vi "resistanceTest.vi"() -> ()   [LabVIEW 2010]
uses:
  <vilib>/DAQmx/read.llb/DAQmx Read (Analog 1D Wfm NChan NSamp).vi
  <vilib>/DAQmx/write.llb/DAQmx Write (Analog DBL 1Chan 1Samp).vi
  <vilib>/daqmx/miscellaneous.llb/DAQmx Fill In Error Info.vi
  <vilib>/ptbypt/NI_PtbyPt.lvlib
panel:
  in  "LowTime":u32
  in  "HighTime":u32
  out "Resistance (MOhm)  2":dbl
  in  "voltage":dbl format="%0.2f"
  out "Test pulse 2":bool
  in  "Test":bool
  out "Numeric 2":i32
  out "Test pulse":bool
  out "Plot":dynamicdata(graph)
  out "stopped":bool
  in  "stop":bool
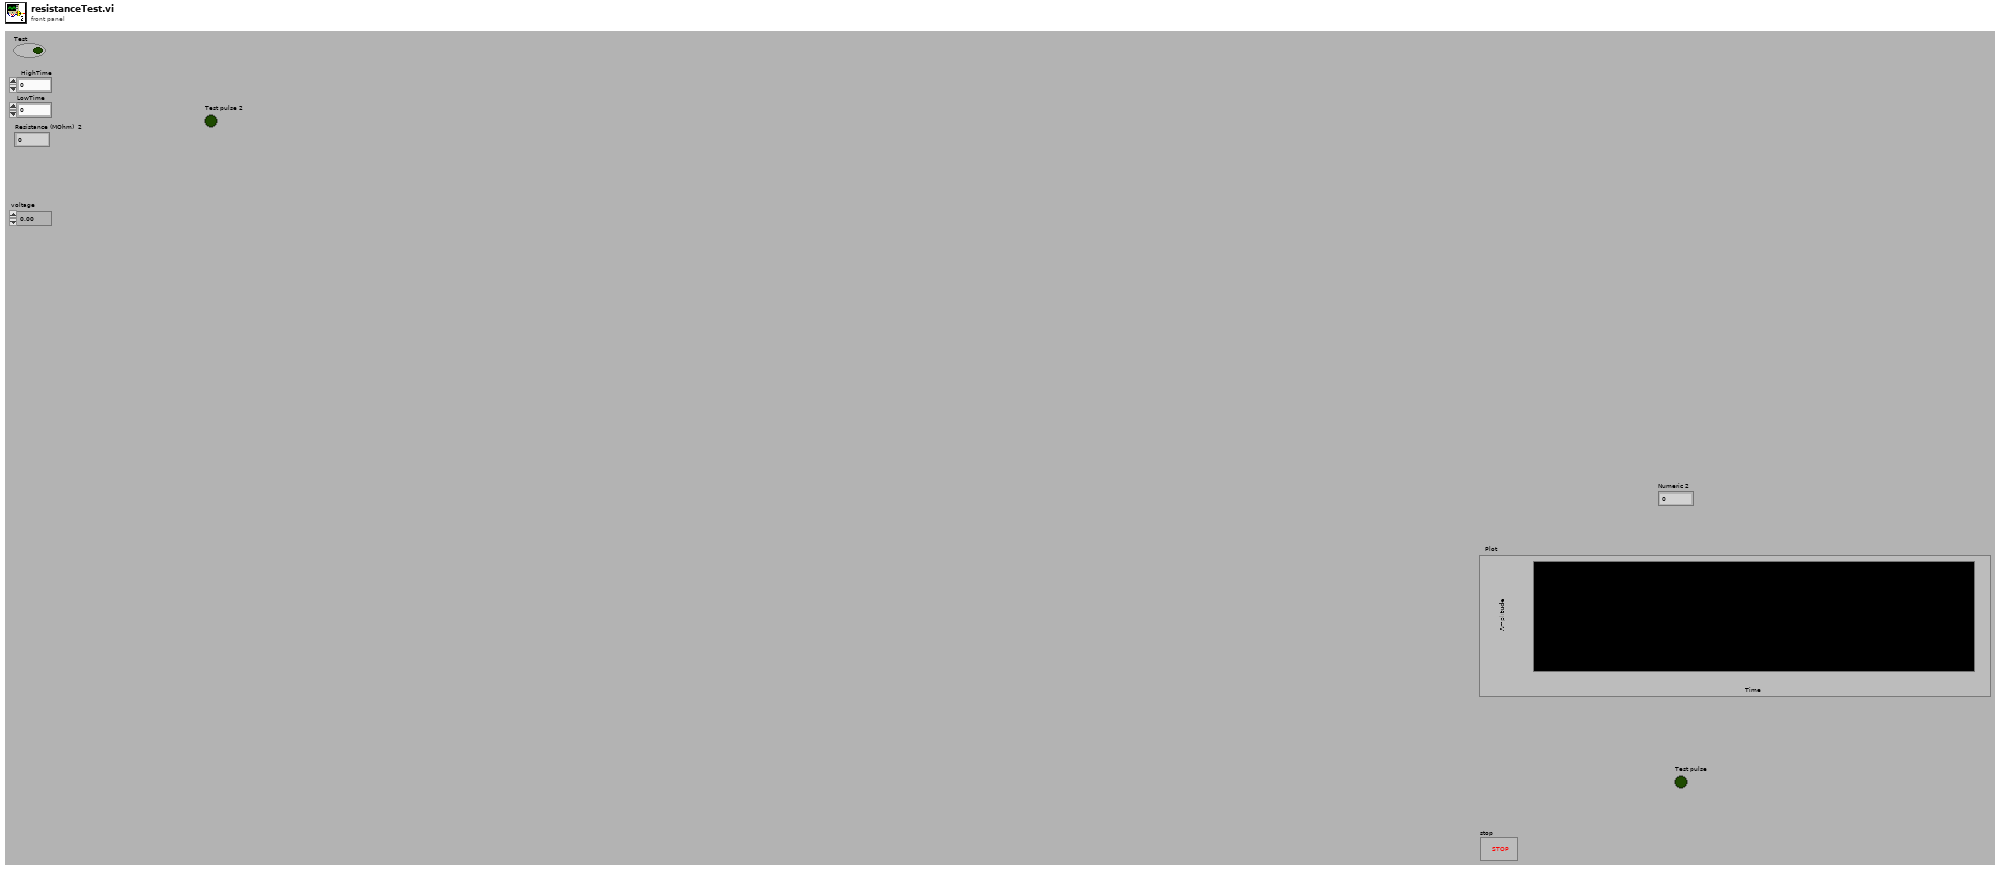
[diagram p1: front panel]
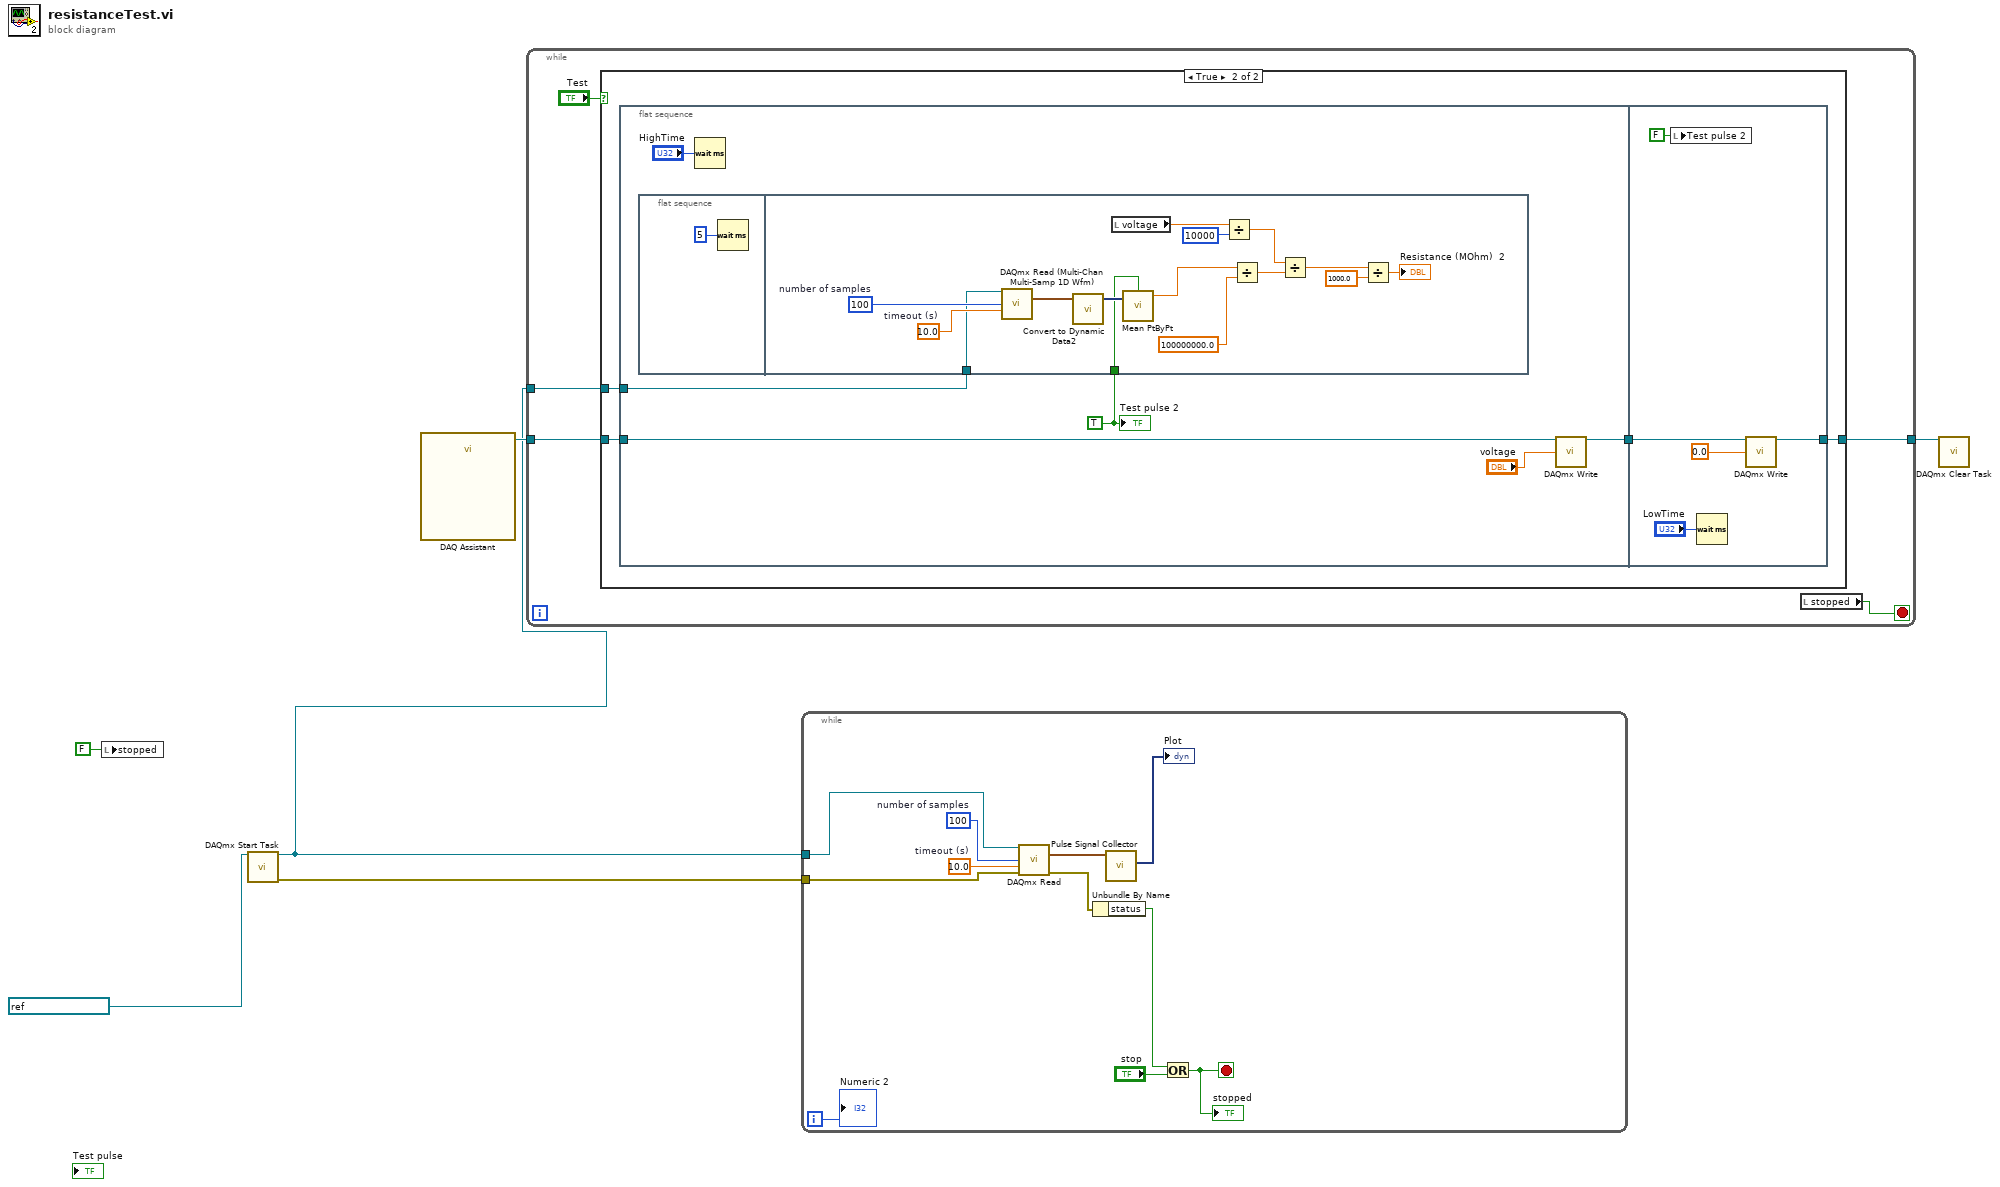
[diagram p0: block diagram]
diagram:
  n1 = local write "stopped"(FALSE ("stopped")) -> ()
  n2 = call <vilib>:"DAQmx Start Task.vi"("task/channels in"=refnum<k21> "ResistanceTest" ("task in")) -> ("task out"=w1:refnum<k21>, "error out"=w5:errorcluster)  [unwired: 13 in]
  n3 = call "DAQ Assistant"() -> ("task out"=w2:refnum<k21>)  [unwired: 18 in, 1 out]
  n4 = while {
    tunnel: w2 -> [w11]
    tunnel: [w10] -> w3
    tunnel: w1 -> [w8]
    stop <- w7 stop-if-true
    n5 = case shown="True" "Test" {
      tunnel: w11 -> [w12 w16]
      tunnel: [w12 w15] -> w10
      tunnel: w8 -> [_ w13]
      frame False {
      }
      frame True {
        n6 = flat-sequence {
          tunnel: w16 -> [w19]
          tunnel: [w20] -> w14
          tunnel: w13 -> [w18]
          tunnel: [w42] -> w15
          tunnel: w14 -> [w39]
          frame #0 {
            w17 = TRUE
            n7 = flat-sequence {
              tunnel: w18 -> [w36]
              tunnel: w17 -> [w33]
              frame #0 {
                n8 = Wait (ms)(milliseconds to wait=u32 5) -> ()  [unwired: 1 out]
              }
              frame #1 {
                w38 = 10.0  # timeout (s)
                w37 = 100  # number of samples
                n9 = call-poly "DAQmx Read (Multi-Chan Multi-Samp 1D Wfm).vi"("task/channels in"=w36, "number of samples per channel"=w37, "timeout"=w38) -> ("data"=w35:waveform(dbl)[])  [unwired: 10 in, 2 out]
                n10 = call "Convert to Dynamic Data2"("Array"=w35) -> ("Dynamic Data Type"=w34:dynamicdata)  [unwired: 3 in]
                n11 = local read "voltage"() -> (w32:dbl)
                n12 = call <vilib>:"Mean PtByPt.vi"("x"=w34, "initialize"=w33) -> ("mean"=w24:dbl)  [unwired: 2 in, 1 out]
                n13 = Divide(x=w32, y=10000) -> (x/y=w27:dbl)
                n14 = Divide(x=w24, y=100000000.0) -> (x/y=w28:dbl)
                n15 = Divide(x=w27, y=w28) -> (x/y=w29:dbl)
                n16 = Divide(x=w29, y=1000.0) -> (x/y=→"Resistance (MOhm)  2":dbl)
              }
            }
            n17 = Wait (ms)(milliseconds to wait="HighTime") -> ()  [unwired: 1 out]
            n18 = call-poly <vilib>:"DAQmx Write.vi"("task/channels in"=w19, "data"="voltage") -> ("task out"=w20:refnum<k21>)  [unwired: 11 in, 2 out]
            "Test pulse 2" <- w17
          }
          frame #1 {
            n19 = local write "Test pulse 2"(FALSE) -> ()
            n20 = Wait (ms)(milliseconds to wait="LowTime") -> ()  [unwired: 1 out]
            n21 = call-poly <vilib>:"DAQmx Write.vi"("task/channels in"=w39, "data"=0.0) -> ("task out"=w42:refnum<k21>)  [unwired: 11 in, 2 out]
          }
        }
      }
    }
    n22 = local read "stopped"() -> (w7:bool)
  }
  n23 = while {
    tunnel: w1 -> [w48]
    tunnel: w5 -> [w49]
    i -> [w44]
    stop <- w47 stop-if-true
    w50 = 10.0  # timeout (s)
    w54 = 100  # number of samples
    n24 = call-poly <vilib>:"DAQmx Read.vi"("task/channels in"=w48, "number of samples per channel"=w54, "timeout"=w50, "error in"=w49) -> ("data"=w45:waveform(dbl)[], "error out"=w53:errorcluster)  [unwired: 9 in, 1 out]
    n25 = Unbundle By Name(w53) -> ("status"=w52:bool)
    n26 = call "Pulse Signal Collector"("Signals"=w45) -> ("Collected Signals"=→"Plot":dynamicdata)  [unwired: 9 in, 1 out]
    n27 = Or(x=w52, y="stop") -> (x .or. y?=w47:bool)
    "stopped" <- w47
    "Numeric 2" <- w44
  }
  n28 = call <vilib>:"DAQmx Clear Task.vi"("task in"=w3) -> ()  [unwired: 14 in, 1 out]
